vi "Section Names Unique.vi"(1 "Section Names":string[](array[string])) -> (0 "Unique?":bool)   [LabVIEW 2012, in "Configuration.lvlib" / "Configuration.lvclass"]
doc: "This VI checks for duplicates in Section Names."
uses:
  Configuration.lvclass
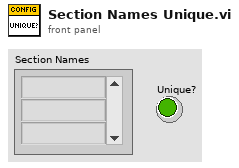
[diagram p1: front panel]
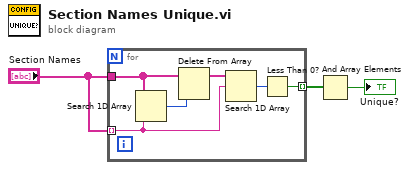
[diagram p0: block diagram]
diagram:
  n1 = for {
    tunnel: "Section Names" -> [w9]
    tunnel: "Section Names" -> [w6] mode=indexing
    tunnel: [w4] -> w2 mode=indexing
    n2 = Search 1D Array(1D array=w9, element=w6) -> (index of element=w8:i32)  [unwired: 1 in]
    n3 = Delete From Array(array=w9, index=w8) -> (array with subset deleted=w7:string[])  [unwired: 1 in, 1 out]
    n4 = Search 1D Array(1D array=w7, element=w6) -> (index of element=w5:i32)  [unwired: 1 in]
    n5 = Less Than 0?(x=w5) -> (x < 0?=w4:bool)
  }
  n6 = And Array Elements(Boolean array=w2) -> (logical AND=→"Unique?":bool)
